vi "set_arbitrary_stimulus.vi"(11 "New stimulus":sgl[][](array[numeric])) -> ()   [LabVIEW 2013]
uses:
  ui_override_opts.ctl
  initialization/micron_globals.vi
panel:
  # "Call this to set the arbitrary stimulus.  Coordinates with update_parameters\nto make sure the stimulus length is updated."
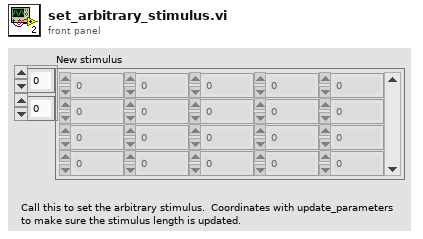
[diagram p1: front panel]
types:
  T1 = typedef "ui_override_opts.ctl" = cluster{"Triggering":bool, "Parameters":bool, "Stimulus":bool, "Calibration":bool, "Modes":bool}
  T2 = typedef "Micron params.ctl" = cluster{"Stimulus":T3, "Goal Filter A":T5, "Mode controls":T6, "Manipulator type":enum16{"Current piezo", "Voltage piezo"}, "Manipulator calibration":T7, "Network":T9, "Goal Filter B":T5, "Cancellation":T10, "Transition time":sgl, "Estimation":T12}
  T3 = typedef "stimulus.ctl" = cluster{"Type":enum16{"Off", "Step", "Sine", "Triangle", "Arbitrary"}, "Phase":dbl, "Amplitude":sgl[], "Injection point":T4, "Closed loop":bool, "Offset":sgl[], "Tip -> world":bool, "Frequency":dbl, "Length":dbl}
  T4 = typedef "injection_point.ctl" = enum16{"Total pose", "V limiter", "Goal ", "Link position", "KF link position", "Inverse kin", "Link goal", "Link error", "Controller", "Output", "Drive", "Light"}
  T5 = typedef "goal_loop_parms.ctl" = cluster{"Speedup max":sgl, "Speedup thresh":sgl, "Speedup nonlin":sgl, "Filters":cluster{"Lower Fc":sgl, "Lower Q":sgl, "Scale factor":sgl, "Upper Fc":sgl, "Upper Q":sgl, "V limit":sgl, "V limit range":sgl}[]}
  T6 = typedef "mode_conrols.ctl" = cluster{"Hold":bool, "Cancellation":bool, "Goal filter":bool, "Trigger":bool}
  T7 = typedef "manipulator_cal.ctl" = cluster{"Tool offsets":sgl[][], "Tip light calibration":T8, "Handle light calibration":T8, "Base pivots":sgl[][], "Output pivots":sgl[][], "Length center":sgl, "Workspace height":sgl[], "Workspace diameter":sgl[], "Linearization":sgl[][], "Stack travel":sgl, "Saturation pos":sgl, "Inverse filters":cluster{"filter structure":enum32{"IIR 2nd Order", "IIR 4th Order"}, "Reverse Coefficients":dbl[], "Forward Coefficients":dbl[]}[]}
  T8 = typedef "probe_calibration.ctl" = sgl[][]
  T9 = typedef "network_params.ctl" = cluster{"Remote Host":string, "Send Status":bool, "Send Port":u16, "Recv Commands":bool, "Recv Port":u16}
  T10 = typedef "sq_control_params.ctl" = cluster{"KP":T11, "KI":sgl, "KD":T11, "Max vel":sgl, "Max acc":sgl, "Int error limit":sgl, "RCM gain":sgl, "Bypass":bool, "Degraded gain":sgl}
  T11 = typedef "decoupled_gain.ctl" = cluster{"XY":sgl, "Rxy":sgl, "Z":sgl, "Rz":sgl}
  T12 = typedef "estimation_controls.ctl" = cluster{"Link":cluster{"Measure noise":dbl[], "Process noise":dbl[], "Alt process noise":dbl[], "Alt turnoff cycles":i32, "Innovation limit":dbl[], "Residue threshold":dbl, "Enable":bool}, "Handle":cluster{"Measure noise":dbl[], "Process noise":dbl[], "State limits":dbl[], "Innovation limit":dbl[], "Prediction Lookahead":sgl, "Enable":bool}}
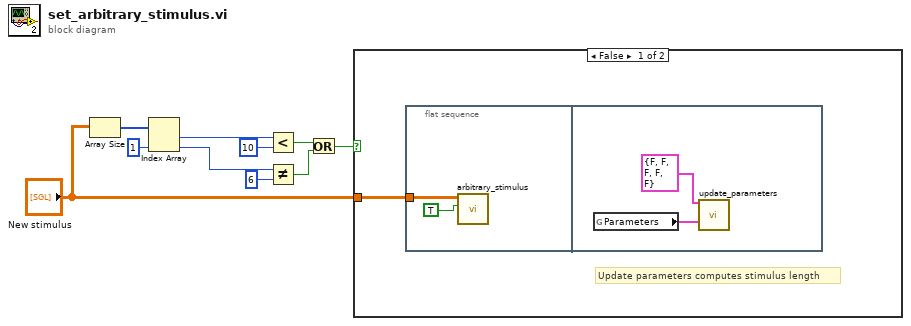
[diagram p0: block diagram]
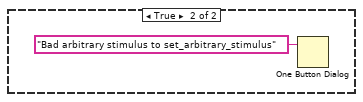
[diagram p2: hidden frame]
diagram:
  n1 = Array Size(array="New stimulus") -> (size(s)=w9:i32[])
  n2 = Index Array(array=w9, index #2=1 ("index")) -> (element #1=w7:i32, element #2=w5:i32)  [unwired: 1 in]
  n3 = Less?(x=w7, y=10) -> (x < y?=w3:bool)
  n4 = Not Equal?(x=w5, y=6) -> (x != y?=w2:bool)
  n5 = Or(x=w3, y=w2) -> (x .or. y?=w1:bool)
  n6 = case shown="False" w1 {
    tunnel: "New stimulus" -> [w11 _]
    frame False {
      # "Update parameters computes stimulus length"
      n7 = flat-sequence {
        tunnel: w11 -> [w12]
        frame #0 {
          n8 = call "arbitrary_stimulus.vi"("Set signal"=TRUE, "New signal"=w12) -> ()  [unwired: 1 in, 9 out]
        }
        frame #1 {
          n9 = global read "micron_globals.vi" "Parameters"() -> (w15:T2)
          n10 = call "update_parameters.vi"("Modify"=T1 {"Triggering"=FALSE, "Parameters"=FALSE, "Stimulus"=FALSE, "Calibration"=FALSE, "Modes"=FALSE}, "Parameters"=w15) -> ()  [unwired: 12 in, 2 out]
        }
      }
    }
    frame True {
      n11 = One Button Dialog(message="Bad arbitrary stimulus to set_arbitrary_stimulus") -> ()  [unwired: 1 in, 1 out]
    }
  }
